vi "Init sync interface.vi"(0 "interface object in":refnum<k20>, 5 "error in (no error)":errorcluster, 8 "node-ID":u8=1) -> (11 "interface object out":refnum<k20>, 14 "TPDO 4 object out":refnum<k20>, 15 "TPDO 3 object out":refnum<k20>, 16 "TPDO 2 object out":refnum<k20>, 17 "TPDO 1 object out":refnum<k20>, 18 "SYNC object out":refnum<k20>, 19 "error out":errorcluster)   [LabVIEW 2016]
uses:
  <vilib>/CANopenLib/CANOPEN.llb/CANopen SYNC Create.vi
  <vilib>/CANopenLib/CANOPEN.llb/CANopen SYNC Start.vi
  <vilib>/CANopenLib/CANOPEN.llb/CANopen TPDO Create.vi
  <vilib>/CANopenLib/CANOPEN.llb/CANopen TPDO Start.vi
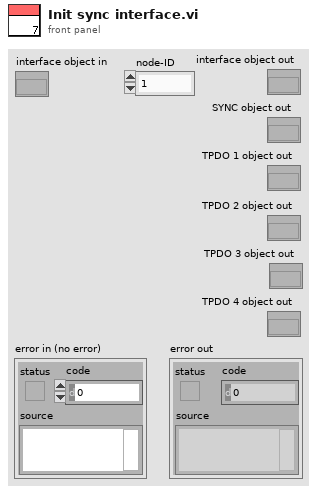
[diagram p1: front panel]
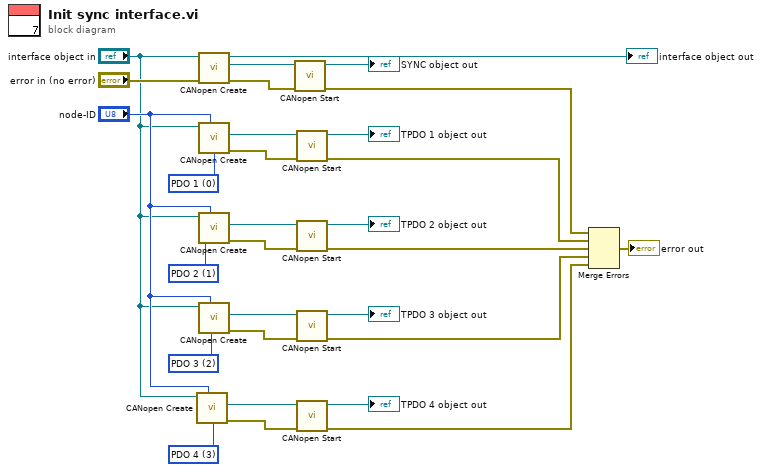
[diagram p0: block diagram]
diagram:
  w16 = u8 3 items=["PDO 1", "PDO 2", "PDO 3", "PDO 4"] ("PDO channel")
  w19 = u8 2 items=["PDO 1", "PDO 2", "PDO 3", "PDO 4"] ("PDO channel")
  w22 = u8 1 items=["PDO 1", "PDO 2", "PDO 3", "PDO 4"] ("PDO channel")
  w25 = u8 0 items=["PDO 1", "PDO 2", "PDO 3", "PDO 4"] ("PDO channel")
  n1 = call-poly <vilib>:"CANopen Create.vi"("node-ID"="node-ID", "PDO channel"=w16, "interface object in"="interface object in") -> ("error out"=w18:errorcluster, "TPDO object out"=w17:refnum<k20>)  [unwired: 6 in, 1 out]
  n2 = call-poly <vilib>:"CANopen Create.vi"("error in (no error)"="error in (no error)", "interface object in"="interface object in") -> ("error out"=w28:errorcluster, "SYNC object out"=w29:refnum<k20>, "interface object out"=→"interface object out":refnum<k20>)  [unwired: 7 in]
  n3 = call-poly <vilib>:"CANopen Create.vi"("node-ID"="node-ID", "PDO channel"=w25, "interface object in"="interface object in") -> ("error out"=w27:errorcluster, "TPDO object out"=w26:refnum<k20>)  [unwired: 6 in, 1 out]
  n4 = call-poly <vilib>:"CANopen Create.vi"("node-ID"="node-ID", "PDO channel"=w22, "interface object in"="interface object in") -> ("error out"=w24:errorcluster, "TPDO object out"=w23:refnum<k20>)  [unwired: 6 in, 1 out]
  n5 = call-poly <vilib>:"CANopen Create.vi"("node-ID"="node-ID", "PDO channel"=w19, "interface object in"="interface object in") -> ("error out"=w21:errorcluster, "TPDO object out"=w20:refnum<k20>)  [unwired: 6 in, 1 out]
  n6 = call-poly <vilib>:"CANopen Start.vi"("error in (no error)"=w28, "SYNC object in"=w29) -> ("error out"=w9:errorcluster, "SYNC object out"=→"SYNC object out":refnum<k20>)  [unwired: 8 in]
  n7 = call-poly <vilib>:"CANopen Start.vi"("error in (no error)"=w27, "TPDO object in"=w26) -> ("error out"=w8:errorcluster, "TPDO object out"=→"TPDO 1 object out":refnum<k20>)  [unwired: 8 in]
  n8 = call-poly <vilib>:"CANopen Start.vi"("error in (no error)"=w24, "TPDO object in"=w23) -> ("error out"=w7:errorcluster, "TPDO object out"=→"TPDO 2 object out":refnum<k20>)  [unwired: 8 in]
  n9 = call-poly <vilib>:"CANopen Start.vi"("error in (no error)"=w21, "TPDO object in"=w20) -> ("error out"=w6:errorcluster, "TPDO object out"=→"TPDO 3 object out":refnum<k20>)  [unwired: 8 in]
  n10 = call-poly <vilib>:"CANopen Start.vi"("error in (no error)"=w18, "TPDO object in"=w17) -> ("error out"=w5:errorcluster, "TPDO object out"=→"TPDO 4 object out":refnum<k20>)  [unwired: 8 in]
  n11 = Merge Errors(w9, w8, w7, w6, w5) -> (→"error out":errorcluster)
